vi "SendNumber - 複製.vi"(2 "Cluster":T1={"試驗速度"=10, "加速時間"=10, "試驗次數"=5000, "輪胎直徑"=660, "異常煞車時間"=50}, 11 "COM Port":refnum<visa-resource-name>="COM6") -> (3 "VISA Output":refnum<visa-resource-name>)   [LabVIEW 2009]
uses:
  <vilib>/Instr/_visa.llb/VISA Configure Serial Port (Instr).vi
panel:
  out "x-y":u32
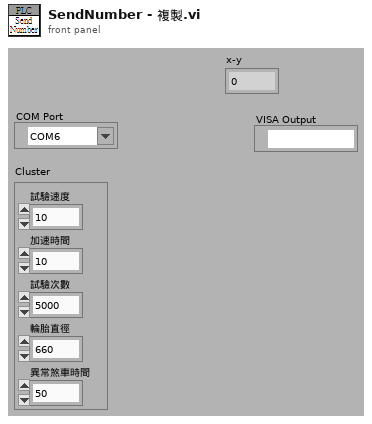
[diagram p1: front panel]
types:
  T1 = cluster{"試驗速度":u32, "加速時間":u32, "試驗次數":u32, "輪胎直徑":u32, "異常煞車時間":u32}
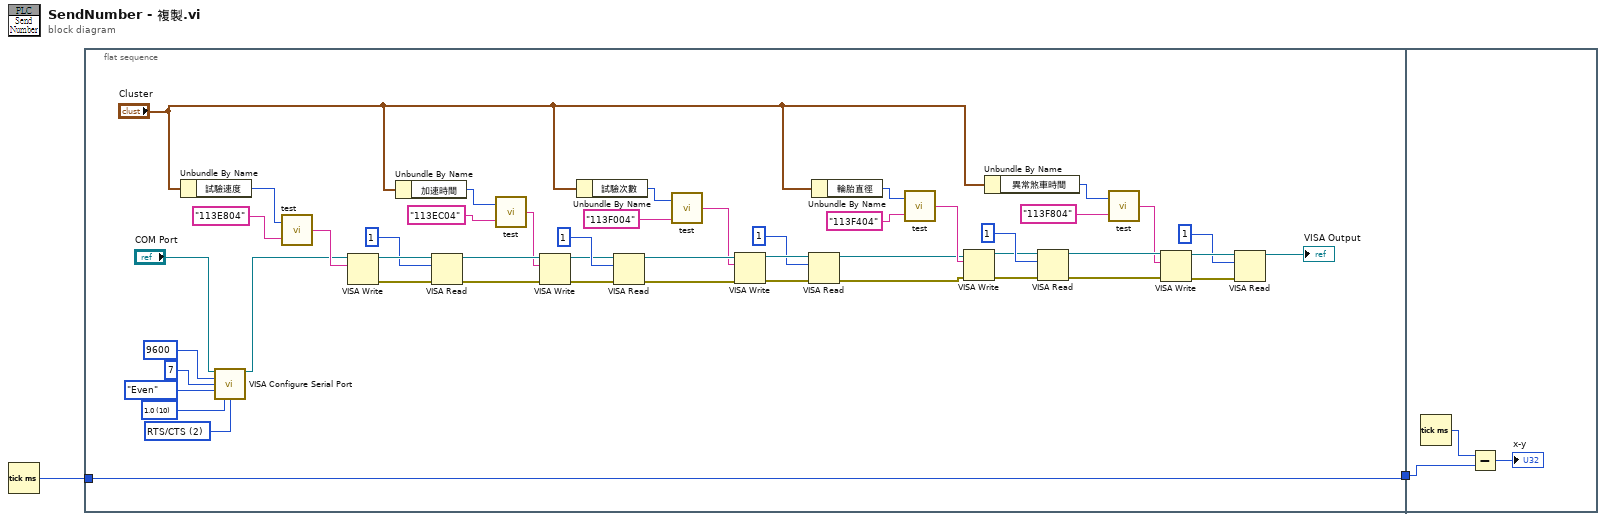
[diagram p0: block diagram]
diagram:
  n1 = Tick Count (ms)() -> (millisecond timer value=w1:u32)
  n2 = flat-sequence {
    tunnel: [w4] -> w2
    tunnel: w1 -> [w4]
    tunnel: w2 -> [w52]
    frame #0 {
      w6 = u16 2 items=["None", "XON/XOFF", "RTS/CTS", "XON/XOFF & RTS/CTS", "DTR/DSR", "XON/XOFF & DTR/DSR"] ("flow control (0:none)")
      w7 = u16 10 items=["1.0"=10, "1.5"=15, "2.0"=20] ("stop bits (10: 1 bit)")
      n3 = Unbundle By Name("Cluster") -> ("試驗速度"=w39:u32)
      n4 = call-poly "VISA Configure Serial Port"("VISA resource name"="COM Port", "baud rate (9600)"=u32 9600, "data bits (8)"=u16 7, "parity (0:none)"=enum16{"None", "Odd", "Even", "Mark", "Space"}."Even", "stop bits (10: 1 bit)"=w7, "flow control (0:none)"=w6) -> ("VISA resource name out"=w5:refnum<visa-resource-name>)  [unwired: 8 in, 1 out]
      n5 = call "test.vi"("String"="113E804", "number"=w39) -> ("concatenated string"=w41:string)
      n6 = VISA Write(VISA resource name=w5, write buffer=w41) -> (VISA resource name out=w49:refnum<visa-resource-name>, error out=w48:errorcluster)  [unwired: 1 in, 1 out]
      n7 = Unbundle By Name("Cluster") -> ("加速時間"=w38:u32)
      n8 = VISA Read(VISA resource name=w49, byte count=u32 1, error in (no error)=w48) -> (VISA resource name out=w43:refnum<visa-resource-name>, error out=w42:errorcluster)  [unwired: 2 out]
      n9 = call "test.vi"("String"="113EC04", "number"=w38) -> ("concatenated string"=w36:string)
      n10 = VISA Write(VISA resource name=w43, write buffer=w36, error in (no error)=w42) -> (VISA resource name out=w44:refnum<visa-resource-name>, error out=w45:errorcluster)  [unwired: 1 out]
      n11 = Unbundle By Name("Cluster") -> ("試驗次數"=w32:u32)
      n12 = VISA Read(VISA resource name=w44, byte count=u32 1, error in (no error)=w45) -> (VISA resource name out=w30:refnum<visa-resource-name>, error out=w29:errorcluster)  [unwired: 2 out]
      n13 = call "test.vi"("String"="113F004", "number"=w32) -> ("concatenated string"=w28:string)
      n14 = VISA Write(VISA resource name=w30, write buffer=w28, error in (no error)=w29) -> (VISA resource name out=w35:refnum<visa-resource-name>, error out=w34:errorcluster)  [unwired: 1 out]
      n15 = VISA Read(VISA resource name=w35, byte count=u32 1, error in (no error)=w34) -> (VISA resource name out=w21:refnum<visa-resource-name>, error out=w20:errorcluster)  [unwired: 2 out]
      n16 = Unbundle By Name("Cluster") -> ("輪胎直徑"=w23:u32)
      n17 = call "test.vi"("String"="113F404", "number"=w23) -> ("concatenated string"=w24:string)
      n18 = VISA Write(VISA resource name=w21, write buffer=w24, error in (no error)=w20) -> (VISA resource name out=w25:refnum<visa-resource-name>, error out=w26:errorcluster)  [unwired: 1 out]
      n19 = Unbundle By Name("Cluster") -> ("異常煞車時間"=w16:u32)
      n20 = VISA Read(VISA resource name=w25, byte count=u32 1, error in (no error)=w26) -> (VISA resource name out=w14:refnum<visa-resource-name>, error out=w12:errorcluster)  [unwired: 2 out]
      n21 = call "test.vi"("String"="113F804", "number"=w16) -> ("concatenated string"=w13:string)
      n22 = VISA Write(VISA resource name=w14, write buffer=w13, error in (no error)=w12) -> (VISA resource name out=w19:refnum<visa-resource-name>, error out=w18:errorcluster)  [unwired: 1 out]
      n23 = VISA Read(VISA resource name=w19, byte count=u32 1, error in (no error)=w18) -> (VISA resource name out=→"VISA Output":refnum<visa-resource-name>)  [unwired: 3 out]
    }
    frame #1 {
      n24 = Tick Count (ms)() -> (millisecond timer value=w53:u32)
      n25 = Subtract(x=w53, y=w52) -> (x-y=→"x-y":u32)
    }
  }
